vi "classify error.vi"(8 "error to classify":errorcluster, 11 "TEC runtime in":refnum<class "TEC runtime.lvclass">) -> (0 "classified error":errorcluster, 2 "error classification":T1, 3 "TEC runtime out":refnum<class "TEC runtime.lvclass">)   [LabVIEW 2013, in "TEC runtime.lvclass"]
doc: "Allows a module to classify an error generated at any point during execution. This <b>error classification</b> can then be used by calling code to determine if execution can continue. In addition, this function can be used to allow a component to clear an error, convert an error to a warning, or attempt to recover from an error. Recovery may be attempted only if <b>attempt recovery?</b> is true."
uses:
  TEC runtime.lvclass
  <vilib>/NI/Tag Bus Module Framework/runtime/error classification.ctl
  <vilib>/NI/Tag Bus Module Framework/runtime/TBM module execution interface.lvclass
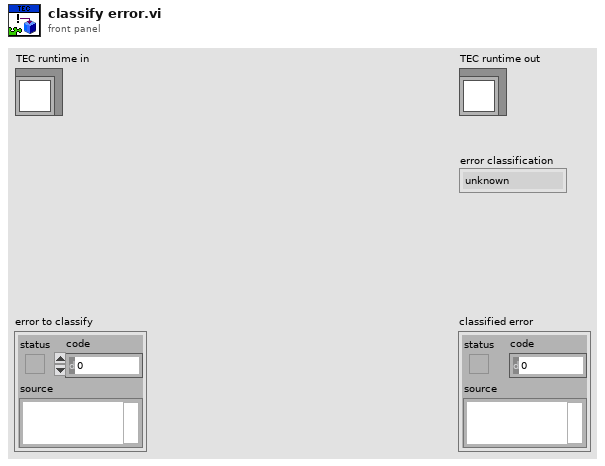
[diagram p1: front panel]
types:
  T1 = typedef "TBM module execution interface.lvclass/error classification.ctl" = enum16{"unknown", "none", "trivial", "recoverable", "critical"}
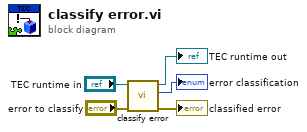
[diagram p0: block diagram]
diagram:
  n1 = call-parent "classify error.vi"("error to classify"="error to classify", "module in"="TEC runtime in") -> ("classified error"=→"classified error":errorcluster, "error classification"=→"error classification":T1, "module out"=→"TEC runtime out":refnum<class "TEC runtime.lvclass">)  [unwired: 7 in]
